vi "Main_Module.vi"(11 "Error_In":errorcluster) -> (15 "Error_Out":errorcluster)   [LabVIEW 2023]
doc: "This is the Main VI for the user to interact with."
uses:
  Controls/Temperature_Limit.ctl
  Controls/Current_Limit.ctl
  Controls/Queue_Operation.ctl
  Controls/Main_Status.ctl
  Controls/Logger_Data.ctl
  Controls/Generated_data.ctl
panel:
  in  "Log_Rate":dbl=1.0 min=1.0 max=120.0
  out "Temperature":dbl
  out "Current":dbl
  out "Generated_Data":dbl[][](graph)
  in  "Exit":bool
  in  "Current_Limit":T1={"Current_High_Limit"=120.0, "Current_Low_Limit"=0.0} caption="Current Limit" {"Current_High_Limit" min=101.0 max=120.0; "Current_Low_Limit" min=100.0 max=119.0}
  in  "Temperature_Limit":T2={"Temperature_High_Limit"=49.0, "Temperature_Low_Limit"=30.0} caption="Temperature Limit" {"Temperature_Low_Limit" min=30.0 max=49.0; "Temperature_High_Limit" min=31.0 max=50.0}
  in  "Start/Stop_Acquisition":bool caption="Start/Stop Acquisition"
  # "ADQ System"
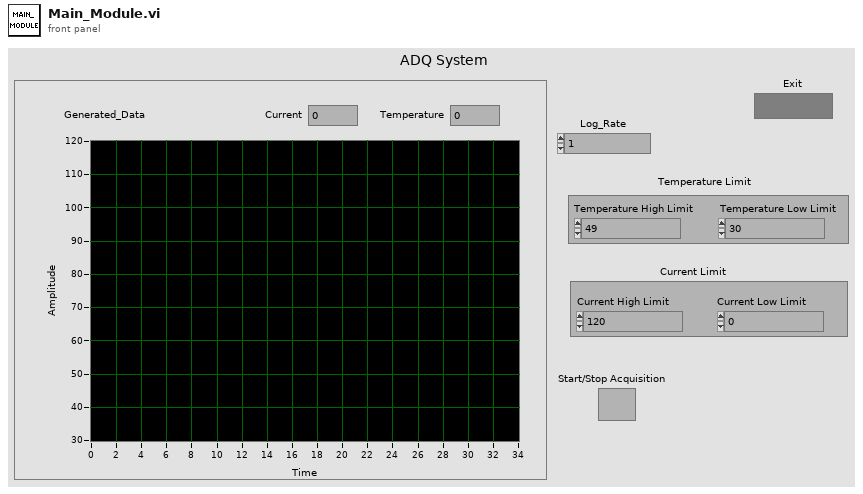
[diagram p1: front panel]
types:
  T1 = typedef "Current_Limit.ctl" = cluster{"Current_High_Limit":dbl, "Current_Low_Limit":dbl}
  T2 = typedef "Temperature_Limit.ctl" = cluster{"Temperature_High_Limit":dbl, "Temperature_Low_Limit":dbl}
  T3 = typedef "Main_Status.ctl" = cluster{"Stop?":bool, "Start/Stop_Acquisition ":bool, "Wait_Time":i32}
  T4 = typedef "Queue_Operation.ctl" = enum16{"Obtain_Queue", "Enqueue", "Lossy_Enqueue", "Preview", "Queue_Status", "Release_Queue", "Dequeue", "Flush"}
  T5 = typedef "Logger_Data.ctl" = cluster{"Generated_Data":T6, "Current_Limit":T1, "Temperature_Limit":T2}
  T6 = typedef "Generated_data.ctl" = cluster{"Current_Data":dbl, "Temp_Data":dbl}
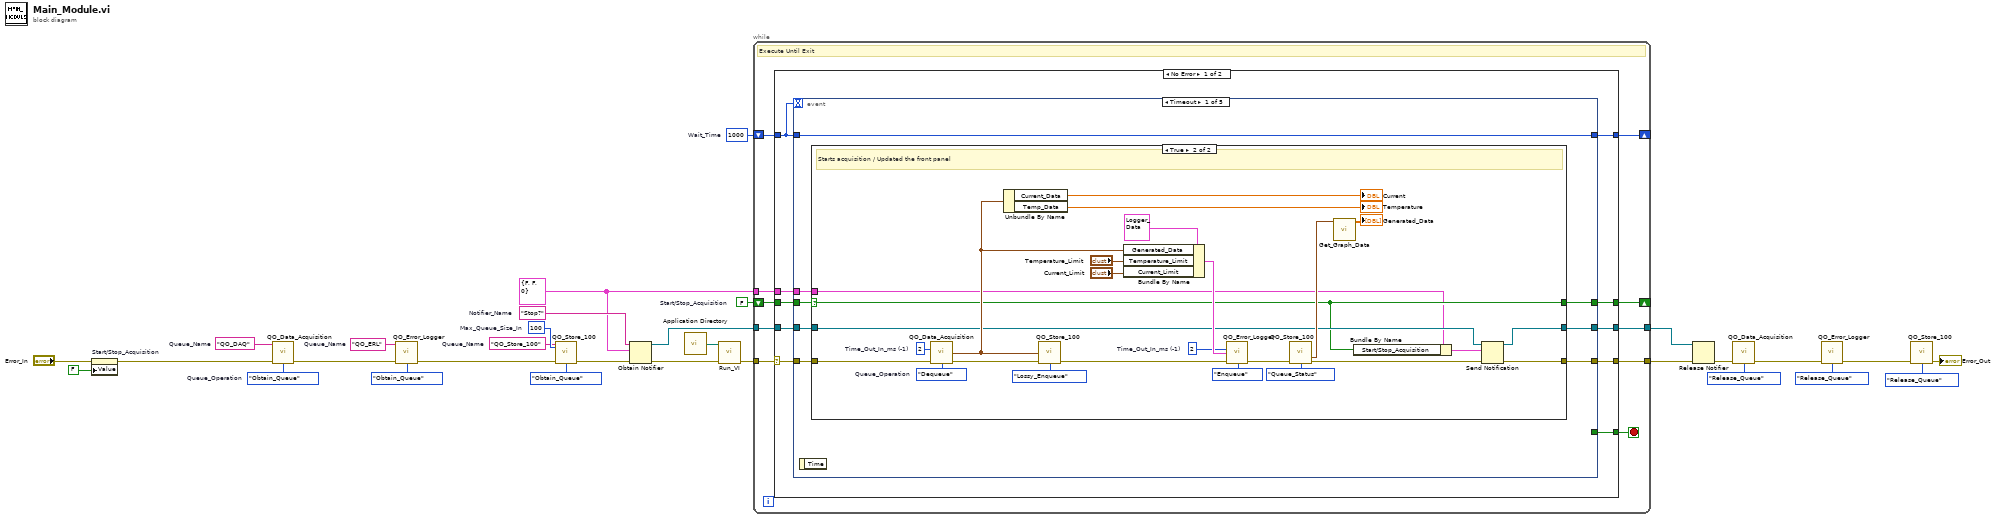
[diagram p0: block diagram]
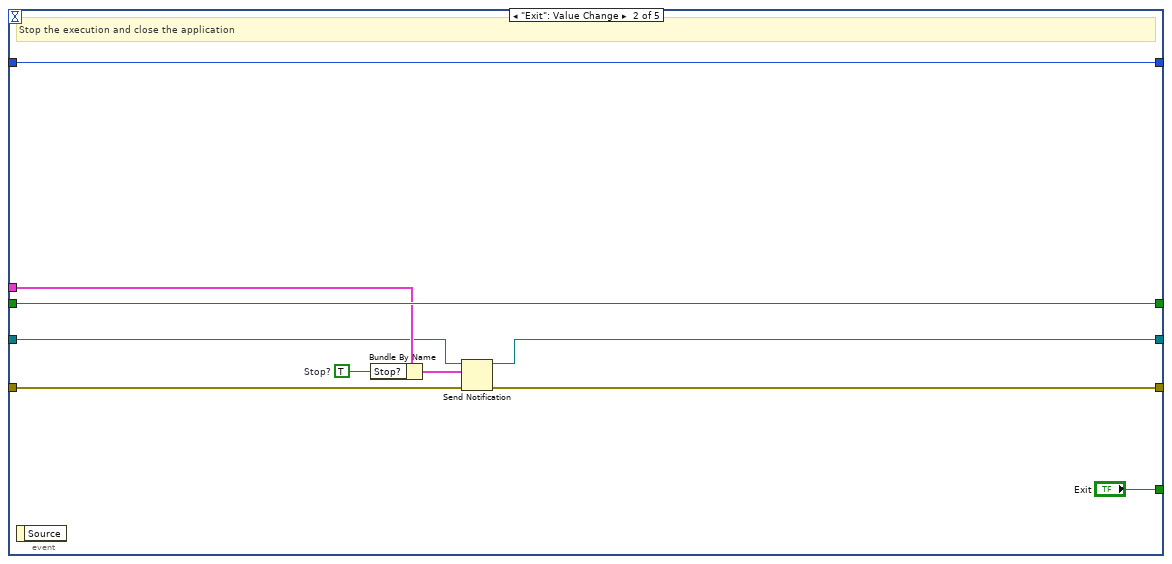
[diagram p3: hidden frame]
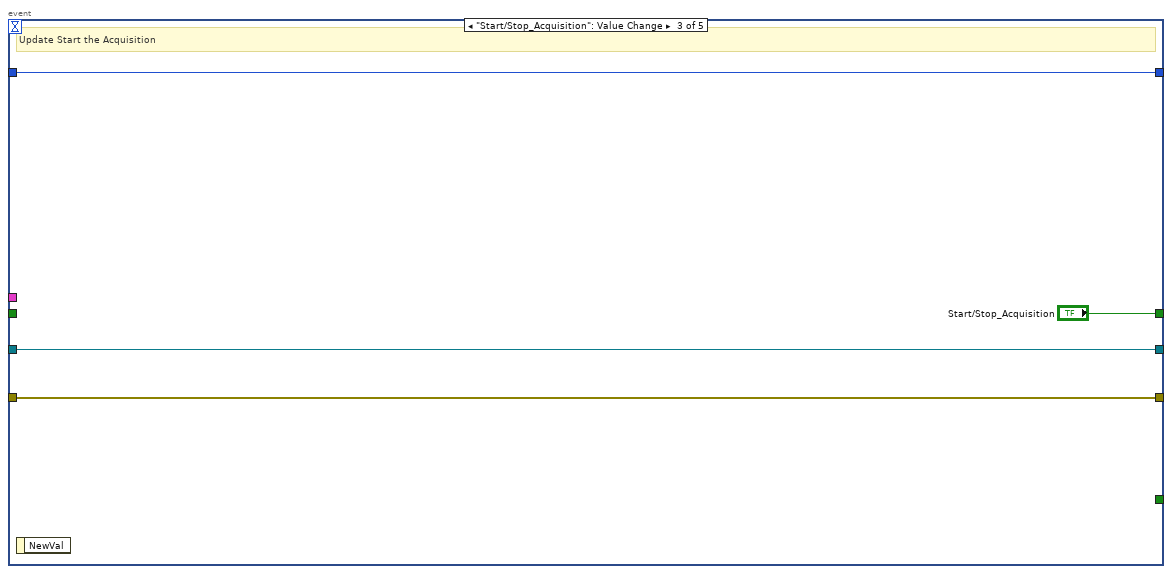
[diagram p4: hidden frame]
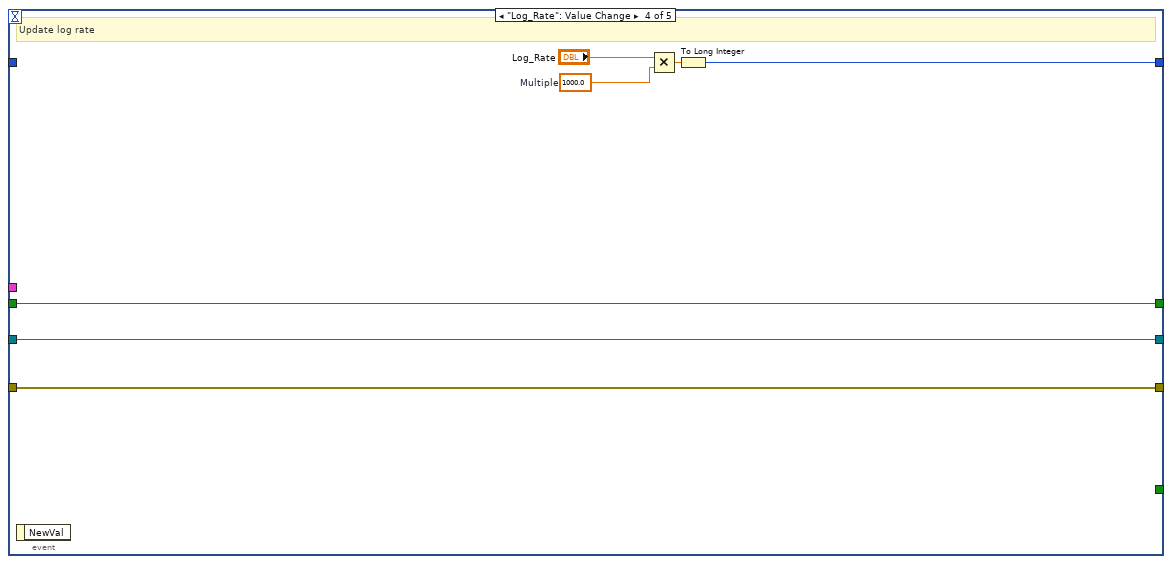
[diagram p5: hidden frame]
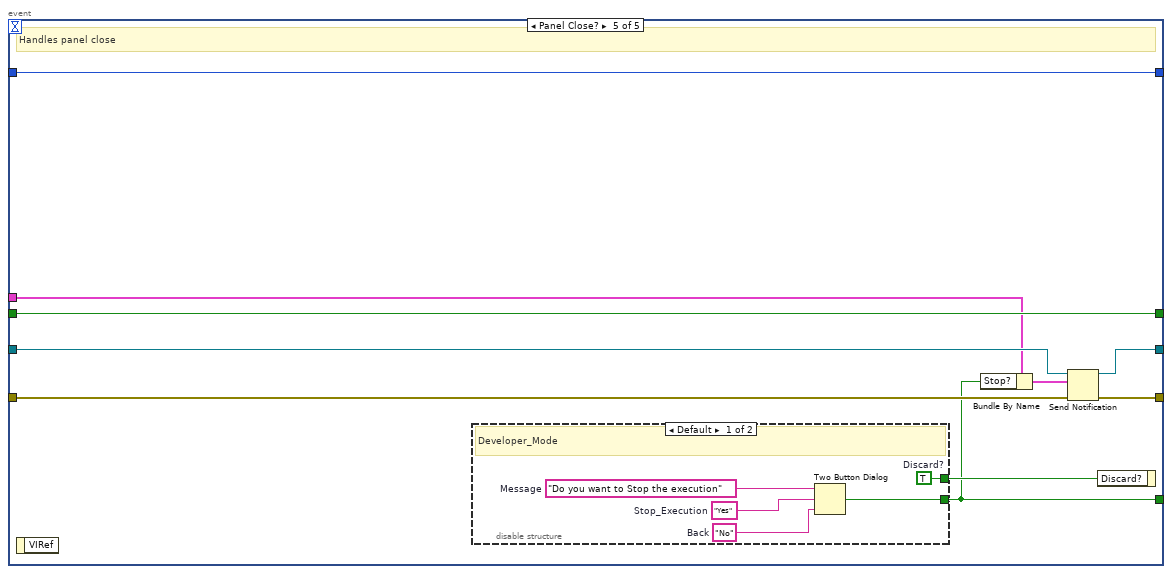
[diagram p6: hidden frame]
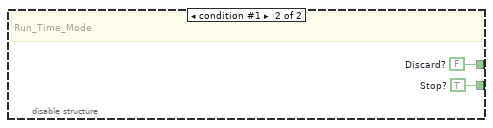
[diagram p7: hidden frame]
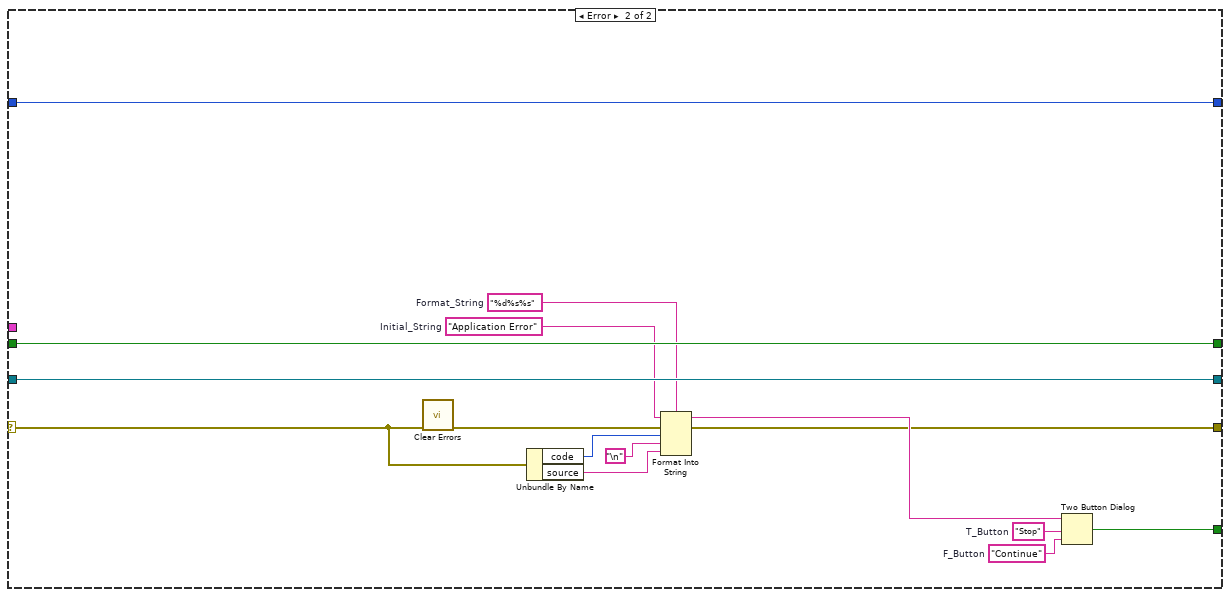
[diagram p8: hidden frame]
diagram:
  w1 = T3 {"Stop?"=FALSE, "Start/Stop_Acquisition "=FALSE, "Wait_Time"=0}
  w10 = "QO_Store_100"  # Queue_Name
  w11 = "QO_ERL"  # Queue_Name
  w12 = "QO_DAQ"  # Queue_Name
  w20 = "Stop?"  # Notifier_Name
  w26 = 1000  # Wait_Time
  w22 = 100  # Max_Queue_Size_In
  w27 = FALSE  # Start/Stop_Acquisition
  w28 = Queue_Operation."Obtain_Queue"  # Queue_Operation
  n1 = property on="Start/Stop_Acquisition" class="Bool (strict)"(error in="Error_In", "Value"=FALSE ("Start/Stop_Acquisition")) -> (error out=w9:errorcluster)  [unwired: 1 in, 1 out]
  n2 = call "QO_Data_Acquisition.vi"("Queue_Name_In"=w12, "Error_In"=w9, "Queue_Operation"=w28) -> ("Error_Out"=w29:errorcluster)  [unwired: 8 in, 4 out]
  n3 = call "QO_Error_Logger.vi"("Queue_Name_In"=w11, "Error_In"=w29, "Queue_Operation"=Queue_Operation."Obtain_Queue") -> ("Error_Out"=w25:errorcluster)  [unwired: 8 in, 4 out]
  n4 = call "QO_Store_100.vi"("Queue_Name_In"=w10, "Max_Queue_Size_In"=w22, "Error_In"=w25, "Queue_Operation"=Queue_Operation."Obtain_Queue") -> ("Error_Out"=w23:errorcluster)  [unwired: 7 in, 4 out]
  n5 = Obtain Notifier(name (unnamed)=w20, notification data type=w1, error in (no error)=w23) -> (notifier out=w19:refnum<notifier>, error out=w16:errorcluster)  [unwired: 1 in, 1 out]
  n6 = call <vilib>:"Application Directory.vi"() -> ("Application Directory"=w14:path)
  n7 = call "Run_VI.vi"("Application_Directory"=w14, "Error_In"=w16) -> ("Error_Out"=w15:errorcluster)  [unwired: 13 in]
  n8 = while {
    tunnel: w15 -> [w40]
    shift-right: [w38] -> _
    shift-left: w27 -> [w37]
    tunnel: [w36] -> w30
    shift-right: [w34] -> _
    shift-left: w26 -> [w35]
    tunnel: w19 -> [w33]
    tunnel: [w32] -> w18
    tunnel: w1 -> [w31]
    stop <- w39 stop-if-true
    # "Execute Until Exit"
    n9 = case shown="No Error" w40 {
      selector: w40 -> [w41 w126]
      tunnel: [w50 w125] -> w39
      tunnel: [w49 w139] -> w38
      tunnel: w37 -> [w48 w139]
      tunnel: [w47 w127] -> w36
      tunnel: w35 -> [w43 w138]
      tunnel: [w46 w138] -> w34
      tunnel: w33 -> [w42 w137]
      tunnel: [w44 w137] -> w32
      tunnel: w31 -> [w45 _]
      frame No Error {
        n10 = event shown="[0] Timeout" {
          selector: _ -> [_ _ _ _ _]
          dyn-events: _ -> [_ _ _ _ _]
          timeout: w43 -> [_ _ _ _ _]
          tunnel: [_ "Exit" _ _ w109] -> w50
          tunnel: [w57 w96 "Start/Stop_Acquisition" w102 w116] -> w49
          tunnel: w48 -> [w56 w96 _ w102 w116]
          tunnel: w41 -> [w54 w95 w101 w104 w115]
          tunnel: [w58 w93 w101 w104 w113] -> w47
          tunnel: [w55 w94 w100 w105 w114] -> w46
          tunnel: w43 -> [w55 w94 w100 _ w114]
          tunnel: w45 -> [w51 w90 _ _ w110]
          tunnel: w42 -> [w53 w89 w98 w103 w112]
          tunnel: [w52 w88 w98 w103 w112] -> w44
          event Timeout {
            n11 = event-data() -> ()  [unwired: 1 in, 1 out]
            n12 = case shown="True" w56 {
              selector: w56 -> [w60 w65]
              tunnel: w54 -> [w61 w87]
              tunnel: [w61 w69] -> w58
              tunnel: [w60 w65] -> w57
              tunnel: w53 -> [w59 w68]
              tunnel: [w59 w67] -> w52
              tunnel: w51 -> [_ w64]
              frame False {
              }
              frame True {
                w71 = 2  # Time_Out_In_ms (-1)
                w72 = 2  # Time_Out_In_ms (-1)
                w86 = Queue_Operation."Dequeue"  # Queue_Operation
                # "Starts acquisition / Updated the front panel"
                n13 = call "QO_Data_Acquisition.vi"("Time_Out_In_ms (-1)"=w72, "Error_In"=w87, "Queue_Operation"=w86) -> ("Data_Out"=w76:T6, "Error_Out"=w84:errorcluster)  [unwired: 8 in, 3 out]
                n14 = Unbundle By Name(w76) -> ("Current_Data"=→"Current":dbl, "Temp_Data"=→"Temperature":dbl)
                n15 = call "QO_Store_100.vi"("Data_In"=w76, "Error_In"=w84, "Queue_Operation"=Queue_Operation."Lossy_Enqueue") -> ("Error_Out"=w73:errorcluster)  [unwired: 8 in, 4 out]
                n16 = Bundle By Name(cluster=T5 {"Generated_Data"={"Current_Data"=0.0, "Temp_Data"=0.0}, "Current_Limit"={"Current_High_Limit"=0.0, "Current_Low_Limit"=0.0}, "Temperature_Limit"={"Temperature_High_Limit"=0.0, "Temperature_Low_Limit"=0.0}} ("Logger_Data"), "Generated_Data"=w76, "Temperature_Limit"="Temperature_Limit", "Current_Limit"="Current_Limit") -> (w78:T5)
                n17 = call "QO_Error_Logger.vi"("Time_Out_In_ms (-1)"=w71, "Data_In"=w78, "Error_In"=w73, "Queue_Operation"=Queue_Operation."Enqueue") -> ("Error_Out"=w80:errorcluster)  [unwired: 7 in, 4 out]
                n18 = call "QO_Store_100.vi"("Error_In"=w80, "Queue_Operation"=Queue_Operation."Queue_Status") -> ("Total_Data"=w81:T6[], "Error_Out"=w70:errorcluster)  [unwired: 9 in, 3 out]
                n19 = call "Get_Graph_Data.vi"("Total_Data"=w81) -> ("Array"=→"Generated_Data":dbl[][])  [unwired: 14 in]
                n20 = Bundle By Name(cluster=w64, "Start/Stop_Acquisition"=w65) -> (w66:T3)
                n21 = Send Notification(notification=w66, notifier=w68, error in (no error)=w70) -> (notifier out=w67:refnum<notifier>, error out=w69:errorcluster)
              }
            }
          }
          event "Exit": Value Change {
            w92 = TRUE  # Stop?
            # "Stop the execution and close the application"
            n22 = event-data() -> ()  [unwired: 1 in, 1 out]
            n23 = Bundle By Name(cluster=w90, "Stop?"=w92) -> (w91:T3)
            n24 = Send Notification(notification=w91, notifier=w89, error in (no error)=w95) -> (notifier out=w88:refnum<notifier>, error out=w93:errorcluster)
          }
          event "Start/Stop_Acquisition": Value Change {
            # "Update Start the Acquisition"
            n25 = event-data() -> ()  [unwired: 1 in, 1 out]
          }
          event "Log_Rate": Value Change {
            w107 = 1000.0  # Multiple
            # "Update log rate"
            n26 = event-data() -> ()  [unwired: 1 in, 1 out]
            n27 = Multiply(x="Log_Rate", y=w107) -> (x*y=w106:dbl)
            n28 = To Long Integer(number=w106) -> (32bit integer=w105:i32)
          }
          event Panel Close? {
            # "Handles panel close"
            n29 = event-data() -> ()  [unwired: 1 in, 1 out]
            n30 = disable-structure shown="Default" {
              disable-tunnel: [w119 w124] -> w109
              disable-tunnel: [w118 w123] -> w117
              frame condition #0 (active) {
                w118 = TRUE  # Discard?
                w120 = "No"  # Back
                w121 = "Yes"  # Stop_Execution
                w122 = "Do you want to Stop the execution"  # Message
                # "Developer_Mode"
                n31 = Two Button Dialog(message=w122, 1:w120, 2:w121) -> (T button?=w119:bool)
              }
              frame condition #1 {
                w123 = FALSE  # Discard?
                w124 = TRUE  # Stop?
                # "Run_Time_Mode"
              }
            }
            n32 = Bundle By Name(cluster=w110, "Stop?"=w109) -> (w111:T3)
            n33 = Send Notification(notification=w111, notifier=w112, error in (no error)=w115) -> (error out=w113:errorcluster)  [unwired: 1 out]
            n34 = event-data("Discard?"=w117) -> ()  [unwired: 1 in, 1 out]
          }
        }
      }
      frame Error {
        w132 = "%d%s%s"  # Format_String
        w133 = "Application Error"  # Initial_String
        w134 = "Stop"  # T_Button
        w135 = "Continue"  # F_Button
        n35 = call <vilib>:"Clear Errors.vi"("error in (no error)"=w126) -> ("error out"=w130:errorcluster)  [unwired: 5 in, 1 out]
        n36 = Unbundle By Name(w126) -> ("code"=w129:i32, "source"=w128:string)
        n37 = Format Into String(format string=w132, initial string=w133, error in=w130, w129, "\n", w128) -> (resulting string=w136:string, error out=w127:errorcluster)
        n38 = Two Button Dialog(message=w136, 1:w135, 2:w134) -> (T button?=w125:bool)
      }
    }
  }
  n39 = Release Notifier(notifier=w18, error in (no error)=w30) -> (error out=w13:errorcluster)  [unwired: 1 in, 2 out]
  n40 = call "QO_Data_Acquisition.vi"("Error_In"=w13, "Queue_Operation"=Queue_Operation."Release_Queue") -> ("Error_Out"=w7:errorcluster)  [unwired: 9 in, 4 out]
  n41 = call "QO_Error_Logger.vi"("Error_In"=w7, "Queue_Operation"=Queue_Operation."Release_Queue") -> ("Error_Out"=w6:errorcluster)  [unwired: 9 in, 4 out]
  n42 = call "QO_Store_100.vi"("Error_In"=w6, "Queue_Operation"=Queue_Operation."Release_Queue") -> ("Error_Out"=→"Error_Out":errorcluster)  [unwired: 9 in, 4 out]
